vi "Page_Version_Initialize.vi"(6 "output cluster":T1, 8 "error in (no error)":errorcluster, 11 "AB_Targetfile in":refnum<class "AB_Targetfile.lvclass">) -> (0 "error out":errorcluster, 3 "AB_Targetfile out":refnum<class "AB_Targetfile.lvclass">)   [LabVIEW 2020, in "AB_Targetfile.lvclass"]
uses:
  <vilib>/AppBuilder/AB_Classes/TargetFile/AB_Targetfile.lvclass
  e:/builds/penguin/labview/branches/2020/dev/dist/vi.lib/AppBuilder/AB_Classes/Build/AB_Build.lvclass
  <resource>/Framework/Providers/Builds/AppBuilder/AB_UI_Page_Version_References.ctl
  <vilib>/AppBuilder/AB_Classes/Build/AB_Build.lvclass
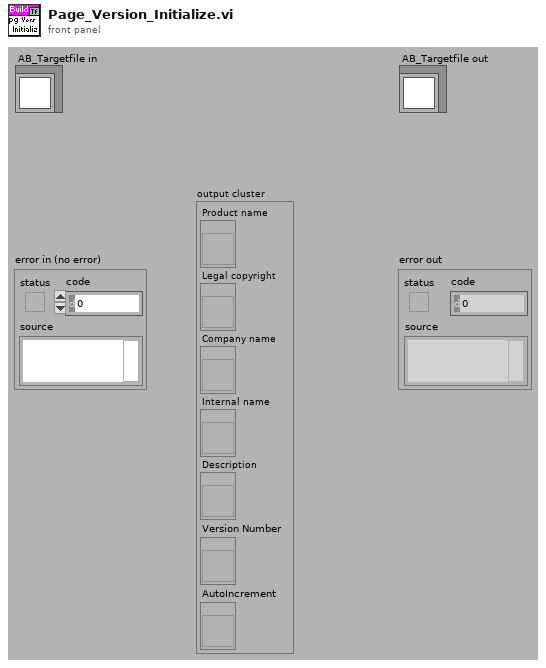
[diagram p1: front panel]
types:
  T1 = typedef "AB_UI_Page_Version_References.ctl" = cluster{"Product name":refnum<vi>, "Legal copyright":refnum<vi>, "Company name":refnum<vi>, "Internal name":refnum<vi>, "Description":refnum<vi>, "Version Number":refnum<vi>, "AutoIncrement":refnum<vi>}
  T2 = enum32{"invalid OS target", "Mac OS", "Windows 3.1", "Windows 95/NT", "Solaris 1", "Solaris 2", "HP-UX", "PowerMAX", "Linux", "Irix", "Rhapsody", "BeOS", "AIX", "OSF1", "VxWorks", "PharLap", "Carbon", "RTX", "Windows x64", "Linux x64", "Mac OS X x64"}
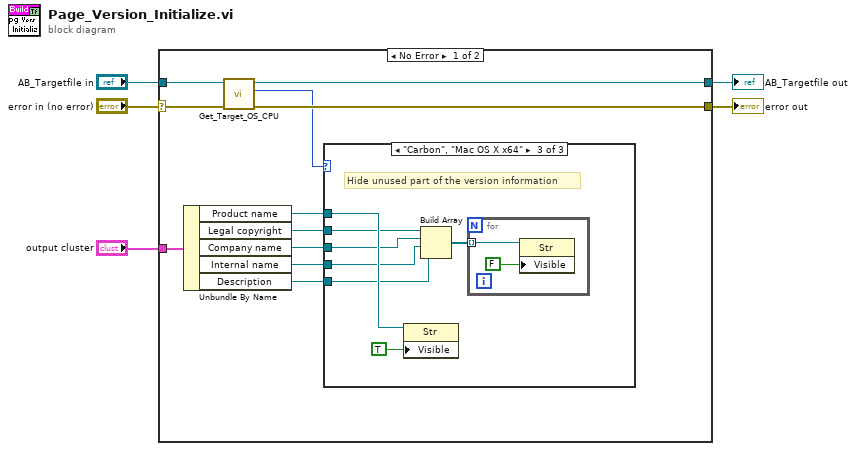
[diagram p0: block diagram]
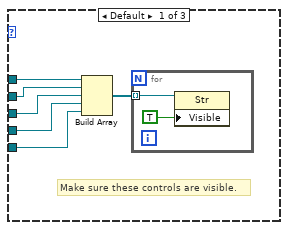
[diagram p2: hidden frame]
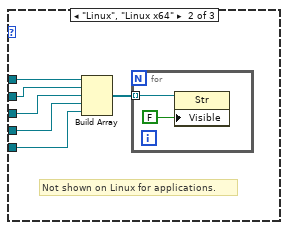
[diagram p3: hidden frame]
diagram:
  n1 = case shown="No Error" "error in (no error)" {
    selector: "error in (no error)" -> [w7 w43]
    tunnel: [w8 w43] -> w2
    tunnel: [w9 w42] -> w4
    tunnel: "AB_Targetfile in" -> [w10 w42]
    tunnel: "output cluster" -> [w16 _]
    frame No Error {
      n2 = Unbundle By Name(w16) -> ("Product name"=w15:refnum<vi>, "Legal copyright"=w13:refnum<vi>, "Company name"=w12:refnum<vi>, "Internal name"=w11:refnum<vi>, "Description"=w14:refnum<vi>)
      n3 = call <vilib>:"Get_Target_OS_CPU.vi"("error in (no error)"=w7, "AB_Build in"=w10) -> ("error out"=w8:errorcluster, "Target Operating System"=w6:T2, "AB_Build out"=w9:refnum<class "AB_Targetfile.lvclass">)  [unwired: 6 in, 1 out]
      n4 = case shown="\"Carbon\", \"Mac OS X x64\"" w6 {
        tunnel: w15 -> [w22 w30 w39]
        tunnel: w14 -> [w18 w26 w33]
        tunnel: w13 -> [w21 w29 w35]
        tunnel: w12 -> [w20 w28 w38]
        tunnel: w11 -> [w19 w27 w34]
        frame Default {
          # "Make sure these controls are visible."
          n5 = Build Array(w22, w21, w20, w19, w18) -> (w17:refnum<vi>[])
          n6 = for {
            tunnel: w17 -> [w23] mode=indexing
            n7 = property class="Str"(reference=w23, "Visible"=TRUE) -> ()  [unwired: 1 in, 2 out]
          }
        }
        frame "Linux", "Linux x64" {
          # "Not shown on Linux for applications."
          n8 = Build Array(w30, w29, w28, w27, w26) -> (w25:refnum<vi>[])
          n9 = for {
            tunnel: w25 -> [w31] mode=indexing
            n10 = property class="Str"(reference=w31, "Visible"=FALSE) -> ()  [unwired: 1 in, 2 out]
          }
        }
        frame "Carbon", "Mac OS X x64" {
          # "Hide unused part of the version information"
          n11 = property class="Str"(reference=w39, "Visible"=TRUE) -> ()  [unwired: 1 in, 2 out]
          n12 = Build Array(w35, w38, w34, w33) -> (w37:refnum<vi>[])
          n13 = for {
            tunnel: w37 -> [w40] mode=indexing
            n14 = property class="Str"(reference=w40, "Visible"=FALSE) -> ()  [unwired: 1 in, 2 out]
          }
        }
      }
    }
    frame Error {
    }
  }
  "error out" <- w2
  "AB_Targetfile out" <- w4
